vi "select ROI select DSF.vi"() -> ()   [LabVIEW 2012]
uses:
  dependencies/LabTIFF/LabTIFF/Opening Purpose.ctl
panel:
  out "error out":errorcluster
  in  "TDSF":i32=2
  in  "downsample?":bool=TRUE
  in  "error in (no error)":errorcluster
  in  "Fish folder Path":path
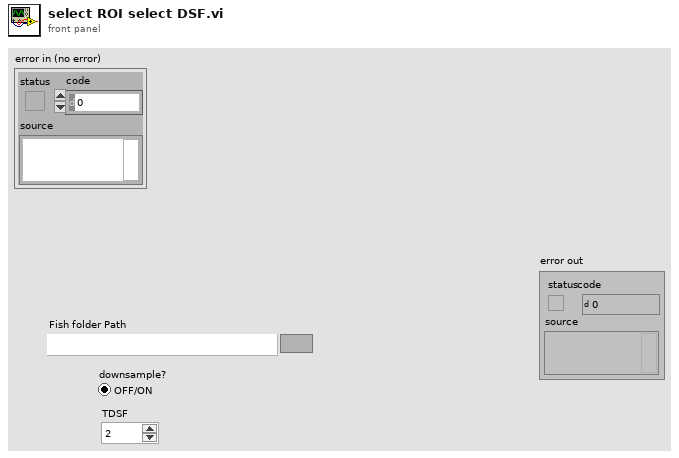
[diagram p1: front panel]
types:
  T1 = typedef "Opening Purpose.ctl" = enum16{"Read", "Write"}
  T2 = enum16{"8 bit unsigned", "16 bit unsigned", "16 bit signed", "32 bit float"}
  T3 = typedef "IMAQ Image.ctl" = refnum<image>
  T4 = typedef "ROI Descriptor" = cluster{"Global Rectangle":i32[], "Contours":cluster{"ID":enum32{"External", "Internal"}, "Type":u32, "Coordinates":i32[]}[]}
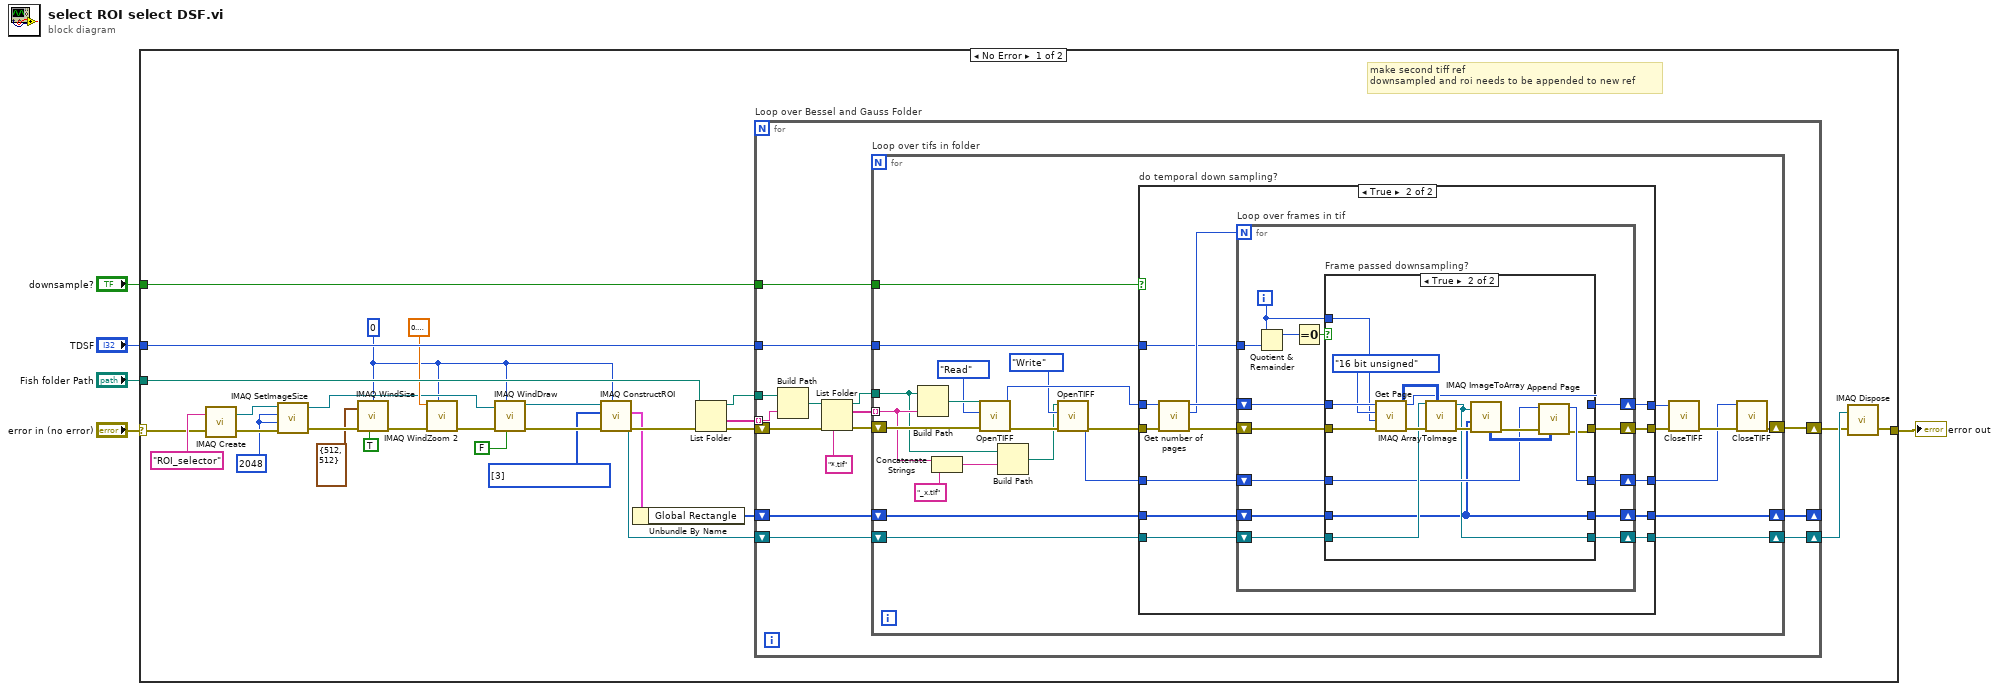
[diagram p0: block diagram]
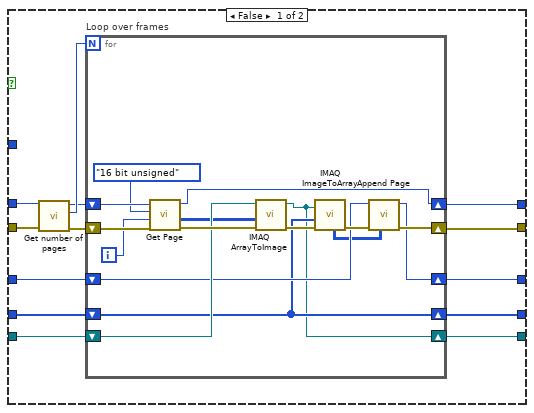
[diagram p2: hidden frame]
diagram:
  n1 = case shown="No Error" "error in (no error)" {
    selector: "error in (no error)" -> [w28 w153]
    tunnel: "Fish folder Path" -> [w27 _]
    tunnel: "downsample?" -> [w32 _]
    tunnel: "TDSF" -> [w31 _]
    tunnel: [w6 w153] -> w1
    frame No Error {
      w14 = u32[] [3] items=["No Selection", "Point", "Line", "Rectangle", "Oval", "Polygon", "Freehand Region", "Annulus", "Zoom", "Pan", "Broken Line", "Freehand Line", "Rotated Rectangle"] ("Tools")
      w13 = 0 ("Window Number")
      w25 = 2048 ("Y Resolution")
      # "make second tiff ref \ndownsampled and roi needs to be appended to new ref"
      n2 = call "IMAQ Create"("Image Name"="ROI_selector", "error in (no error)"=w28) -> ("New Image"=w26:T3, "error out"=w30:errorcluster)  [unwired: 3 in]
      n3 = call "IMAQ SetImageSize"("error in (no error)"=w30, "Y Resolution"=w25, "X Resolution"=w25, "Image"=w26) -> ("error out"=w20:errorcluster, "Image Out"=w18:T3)  [unwired: 1 in]
      n4 = call "IMAQ WindSize"("error in (no error)"=w20, "Get/Set Status? (Set)"=TRUE, "Width & Height"=cluster{"Width":i32, "Height":i32} {"Width"=512, "Height"=512}, "Window Number"=w13) -> ("error out"=w21:errorcluster)  [unwired: 2 in, 2 out]
      n5 = call "IMAQ WindZoom 2"("Window Number (0...15)"=w13, "error in (no error)"=w21, "Zoom Factor"=sgl 0.2) -> ("error out"=w22:errorcluster)  [unwired: 5 in, 3 out]
      n6 = call "IMAQ WindDraw"("Resize to Image Size? (Y)"=FALSE, "Window Number (0...15)"=w13, "error in (no error)"=w22, "Image"=w18) -> ("error out"=w16:errorcluster, "Image Out (duplicate)"=w15:T3)  [unwired: 6 in]
      n7 = call "IMAQ ConstructROI"("Window Number (-1...15)"=w13, "error in (no error)"=w16, "Tools"=w14, "Image"=w15) -> ("error out"=w12:errorcluster, "ROI Descriptor Out"=w10:T4, "Image Out (duplicate)"=w11:T3)  [unwired: 4 in, 1 out]
      n8 = Unbundle By Name(w10) -> ("Global Rectangle"=w9:i32[])
      n9 = List Folder(path=w27, error in=w12) -> (path out=w33:path, folder names=w34:string[], error out=w35:errorcluster)  [unwired: 2 in, 1 out]
      n10 = for "Loop over Bessel and Gauss Folder" {
        tunnel: w34 -> [w49] mode=indexing
        tunnel: w33 -> [w50]
        tunnel: w32 -> [w42]
        shift-right: [w40] -> w7
        shift-left: w35 -> [w46]
        tunnel: w31 -> [w41]
        shift-right: [w37] -> w8
        shift-left: w11 -> [w39]
        shift-right: [w36] -> _
        shift-left: w9 -> [w38]
        n11 = Build Path(base path=w50, name or relative path=w49) -> (appended path=w47:path)
        n12 = List Folder(path=w47, pattern="*.tif", error in=w46) -> (path out=w43:path, filenames=w44:string[], error out=w45:errorcluster)  [unwired: 1 in, 1 out]
        n13 = for "Loop over tifs in folder" {
          tunnel: w44 -> [w62] mode=indexing
          tunnel: w43 -> [w59]
          tunnel: w42 -> [w70]
          shift-right: [w56] -> w40
          shift-left: w45 -> [w74]
          tunnel: w41 -> [w69]
          shift-right: [w52] -> w37
          shift-left: w39 -> [w68]
          shift-right: [w51] -> w36
          shift-left: w38 -> [w67]
          n14 = Build Path(base path=w59, name or relative path=w62) -> (appended path=w73:path)
          n15 = Concatenate Strings(w62, "_x.tif" ("string")) -> (w60:string)
          n16 = call "OpenTIFF.vi"("error in (no error)"=w74, "Opening Purpose"=Opening_Purpose."Read", "File Path"=w73) -> ("error out"=w66:errorcluster, "TIFF File Ref"=w71:i32)  [unwired: 7 in]
          n17 = Build Path(base path=w59, name or relative path=w60) -> (appended path=w58:path)
          n18 = call "OpenTIFF.vi"("error in (no error)"=w66, "Opening Purpose"=Opening_Purpose."Write", "File Path"=w58) -> ("error out"=w65:errorcluster, "TIFF File Ref"=w64:i32)  [unwired: 7 in]
          n19 = case "do temporal down sampling?" shown="True" w70 {
            tunnel: w65 -> [w87 w117]
            tunnel: w71 -> [w86 w115]
            tunnel: w69 -> [_ w112]
            tunnel: [w79 w111] -> w55
            tunnel: w68 -> [w81 w110]
            tunnel: w67 -> [w82 w109]
            tunnel: w64 -> [w80 w108]
            tunnel: [w78 w106] -> w54
            tunnel: [w77 w107] -> w53
            tunnel: [w75 w105] -> w52
            tunnel: [w76 w104] -> w51
            frame False {
              n20 = call "Get number of pages.vi"("error in (no error)"=w87, "TIFF File ref"=w86) -> ("error out"=w85:errorcluster, "Number of Pages"=w84:i32, "TIFF File ref out"=w83:i32)  [unwired: 7 in]
              n21 = for "Loop over frames" {
                N: w84 -> [_]
                shift-right: [w96] -> w79
                shift-left: w85 -> [w103]
                shift-right: [w93] -> w77
                shift-left: w83 -> [w102]
                shift-right: [w90] -> w76
                shift-left: w82 -> [w90]
                shift-right: [w89] -> w78
                shift-left: w80 -> [w92]
                shift-right: [w88] -> w75
                shift-left: w81 -> [w95]
                i -> [w101]
                n22 = call "Get Page.vi"("error in (no error)"=w103, "Frame number"=w101, "Type of Image"=T2."16 bit unsigned", "TIFF File Ref"=w102) -> ("error out"=w99:errorcluster, "U16 Image out"=w94:u16[][], "TIFF File Ref out"=w93:i32)  [unwired: 2 in, 3 out]
                n23 = call "IMAQ ArrayToImage"("Image Pixels (U16)"=w94, "error in (no error)"=w99, "Image"=w95) -> ("error out"=w98:errorcluster, "Image Out"=w88:T3)  [unwired: 7 in]
                n24 = call "IMAQ ImageToArray"("error in (no error)"=w98, "Optional Rectangle"=w90, "Image"=w88) -> ("Image Pixels (U16)"=w91:u16[][], "error out"=w97:errorcluster)  [unwired: 1 in, 3 out]
                n25 = call "Append Page.vi"("U16 Image"=w91, "error in (no error)"=w97, "TIFF File Ref"=w92) -> ("error out"=w96:errorcluster, "TIFF File Ref out"=w89:i32)  [unwired: 7 in]
              }
            }
            frame True {
              n26 = call "Get number of pages.vi"("error in (no error)"=w117, "TIFF File ref"=w115) -> ("error out"=w116:errorcluster, "Number of Pages"=w113:i32, "TIFF File ref out"=w114:i32)  [unwired: 7 in]
              n27 = for "Loop over frames in tif" {
                N: w113 -> [_]
                shift-right: [w125] -> w111
                shift-left: w116 -> [w128]
                tunnel: w112 -> [w131]
                shift-right: [w124] -> w107
                shift-left: w114 -> [w127]
                shift-right: [w119] -> w105
                shift-left: w110 -> [w123]
                shift-right: [w118] -> w104
                shift-left: w109 -> [w122]
                shift-right: [w120] -> w106
                shift-left: w108 -> [w121]
                i -> [w126]
                n28 = Quotient & Remainder(x=w126, y=w131) -> (x-y*floor(x/y)=w130:i32)  [unwired: 1 out]
                n29 = Equal To 0?(x=w130) -> (x = 0?=w129:bool)
                n30 = case "Frame passed downsampling?" shown="True" w129 {
                  tunnel: w128 -> [w136 w152]
                  tunnel: w127 -> [w135 w151]
                  tunnel: w126 -> [_ w149]
                  tunnel: [w136 w139] -> w125
                  tunnel: [w135 w140] -> w124
                  tunnel: w123 -> [w134 w146]
                  tunnel: w122 -> [w133 w137]
                  tunnel: w121 -> [w132 w142]
                  tunnel: [w132 w141] -> w120
                  tunnel: [w134 w138] -> w119
                  tunnel: [w133 w137] -> w118
                  frame False {
                  }
                  frame True {
                    n31 = call "Get Page.vi"("error in (no error)"=w152, "Frame number"=w149, "Type of Image"=T2."16 bit unsigned", "TIFF File Ref"=w151) -> ("error out"=w148:errorcluster, "U16 Image out"=w147:u16[][], "TIFF File Ref out"=w140:i32)  [unwired: 2 in, 3 out]
                    n32 = call "IMAQ ArrayToImage"("Image Pixels (U16)"=w147, "error in (no error)"=w148, "Image"=w146) -> ("error out"=w145:errorcluster, "Image Out"=w138:T3)  [unwired: 7 in]
                    n33 = call "IMAQ ImageToArray"("error in (no error)"=w145, "Optional Rectangle"=w137, "Image"=w138) -> ("Image Pixels (U16)"=w144:u16[][], "error out"=w143:errorcluster)  [unwired: 1 in, 3 out]
                    n34 = call "Append Page.vi"("U16 Image"=w144, "error in (no error)"=w143, "TIFF File Ref"=w142) -> ("error out"=w139:errorcluster, "TIFF File Ref out"=w141:i32)  [unwired: 7 in]
                  }
                }
              }
            }
          }
          n35 = call "CloseTIFF.vi"("error in (no error)"=w55, "TIFF File Ref"=w53) -> ("error out"=w57:errorcluster)  [unwired: 9 in]
          n36 = call "CloseTIFF.vi"("error in (no error)"=w57, "TIFF File Ref"=w54) -> ("error out"=w56:errorcluster)  [unwired: 9 in]
        }
      }
      n37 = call "IMAQ Dispose"("Image"=w8, "error in (no error)"=w7) -> ("error out"=w6:errorcluster)  [unwired: 4 in]
    }
    frame Error {
    }
  }
  "error out" <- w1
